vi "Generate AC Measurement Waveform Multi Channel.vi"(6 "hardware commands sync queue":T1, 7 "Voltage(volts)":dbl, 8 "error in":errorcluster, 9 "Frequency":dbl, 10 "DAQmx product name":string, 11 "DSG task in":refnum<k21>) -> (0 "error out":errorcluster, 3 "DSG task out":refnum<k21>)   [LabVIEW 2021, in "audio_adc_acDualChannelMeasurement.lvlib"]
uses:
  audio_adc_acDualChannelMeasurement.lvlib
  shared/controls/Sync Commands Queue Ref.ctl
  shared/controls/Sync Commands.ctl
  <vilib>/addons/_NISVFA/_Generation/Signal Generation/SV Signal/sv_System Timing Model.ctl
  <vilib>/DAQmx/write.llb/DAQmx Write (Analog 1D Wfm NChan NSamp).vi
  <vilib>/addons/_NISVFA/_Generation/Signal Generation/SV Sinusoid/SV Sinusoid.lvclass
  C:/Program Files/National Instruments/LabVIEW 2021/vi.lib/addons/_NISVFA/_Generation/Signal Generation/SV Signal/SV Signal.lvclass
  <vilib>/addons/_NISVFA/_Generation/Signal Generation/SV Sinusoid/Configure Sine.vi
  <vilib>/addons/_NISVFA/_Generation/Signal Generation/SV Signal/Write Sample Rate.vi
  <vilib>/addons/_NISVFA/_Generation/Signal Generation/SV Signal/Write System Timing Model.vi
  <vilib>/addons/_NISVFA/_Generation/Signal Generation/SV Signal/Write Ramp Parameters.vi
  <vilib>/DAQmx/miscellaneous.llb/DAQmx Fill In Error Info.vi
  <resource>/objmgr/daqmx.rc
  <vilib>/addons/_NISVFA/_Generation/Signal Generation/SV Signal/SV Signal.lvclass
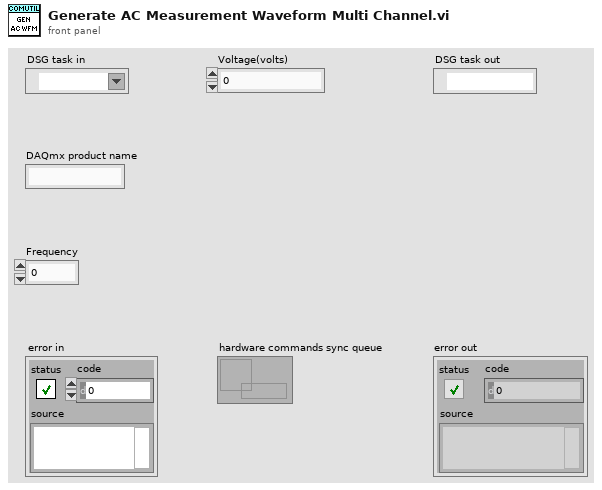
[diagram p1: front panel]
types:
  T1 = typedef "Sync Commands Queue Ref.ctl" = refnum<queue>
  T2 = typedef "Sync Commands.ctl" = enum16{"NoAction", "GenerationStarted", "AcquisitionCompleted", "GenerationErrored"}
  T3 = cluster{"profile":enum16{"Linear", "Half cosine"}, "durations [s]":cluster{"ramp-up":dbl, "transition":dbl, "ramp-down":dbl}}
  T4 = typedef "SV Signal.lvclass/sv_System Timing Model.ctl" = i64
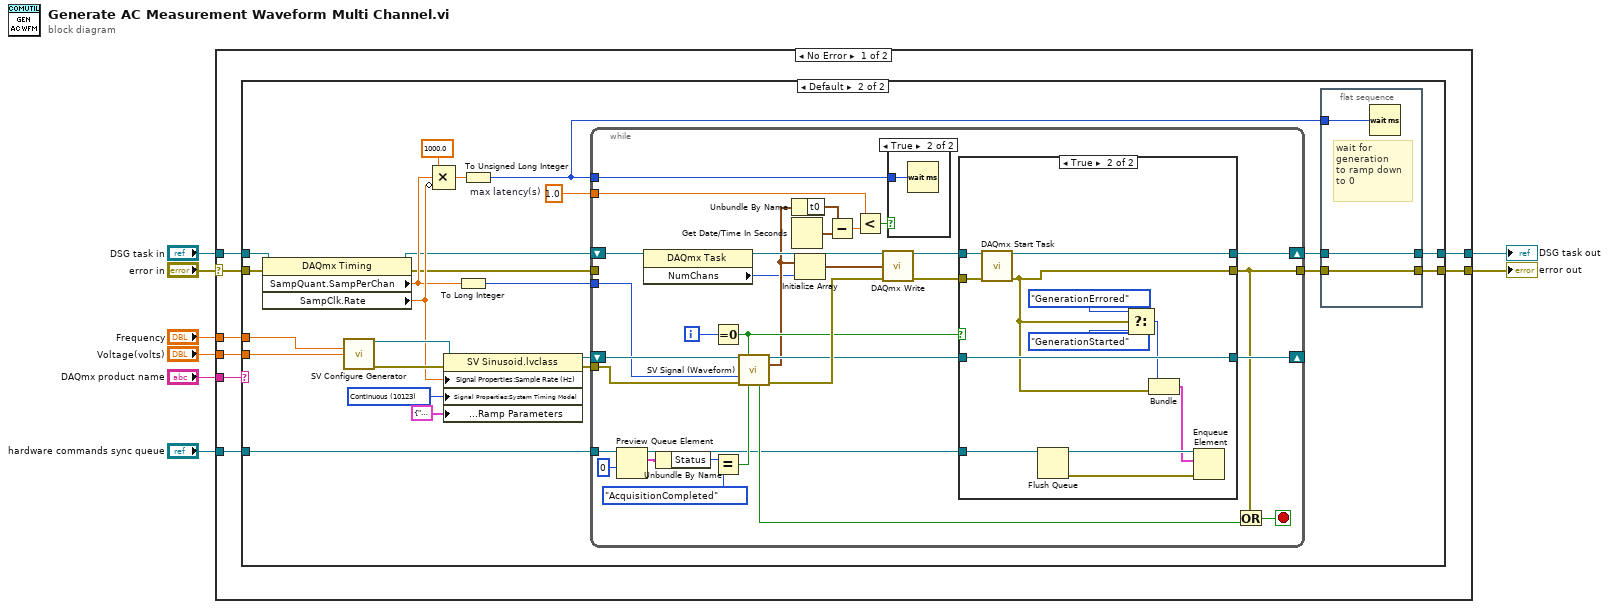
[diagram p0: block diagram]
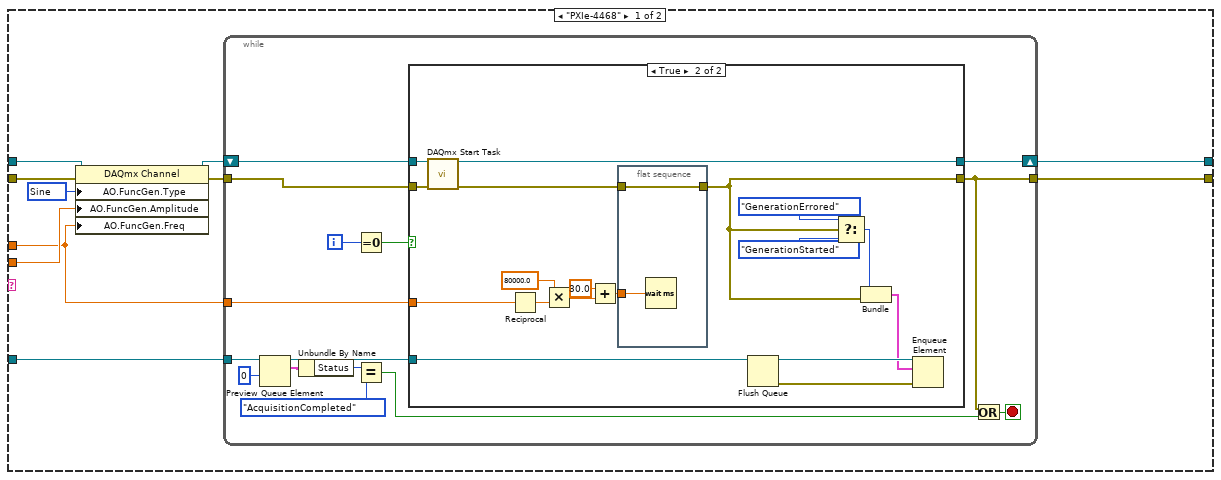
[diagram p2: hidden frame]
diagram:
  n1 = case shown="No Error" "error in" {
    selector: "error in" -> [w16 w140]
    tunnel: [w15 w139] -> w7
    tunnel: [w14 w140] -> w6
    tunnel: "DSG task in" -> [w11 w139]
    tunnel: "hardware commands sync queue" -> [w13 _]
    tunnel: "DAQmx product name" -> [w10 _]
    tunnel: "Frequency" -> [w9 _]
    tunnel: "Voltage(volts)" -> [w12 _]
    frame No Error {
      n2 = case shown="Default" w10 {
        tunnel: w16 -> [w20 w87]
        tunnel: w11 -> [w22 w83]
        tunnel: [w25 w71] -> w15
        tunnel: [w24 w70] -> w14
        tunnel: w13 -> [w26 w68]
        tunnel: w9 -> [w17 w66]
        tunnel: w12 -> [w18 w65]
        frame "PXIe-4468" {
          w19 = 14751 items=["Sine"=14751, "Triangle"=14752, "Square"=14753, "Sawtooth"=14754] ("AO.FuncGen.Type")
          n3 = property class="DAQmx Channel"(reference=w22, error in=w20, "AO.FuncGen.Type"=w19, "AO.FuncGen.Amplitude"=w18, "AO.FuncGen.Freq"=w17) -> (reference out=w23:refnum<k21>, error out=w21:errorcluster)
          n4 = while {
            tunnel: w21 -> [w40]
            shift-right: [w34] -> w25
            shift-left: w23 -> [w39]
            tunnel: [w27] -> w24
            tunnel: w26 -> [w31]
            tunnel: w17 -> [w28]
            i -> [w41]
            stop <- w38 stop-if-true
            n5 = Preview Queue Element(queue=w31, timeout in ms (-1)=0) -> (queue out=w35:T1, element=w33:cluster{"Status":T2, "Error":errorcluster})  [unwired: 1 in, 2 out]
            n6 = Unbundle By Name(w33) -> ("Status"=w32:T2)
            n7 = Equal To 0?(x=w41) -> (x = 0?=w30:bool)
            n8 = Equal?(x=w32, y=Sync_Commands."AcquisitionCompleted") -> (x = y?=w29:bool)
            n9 = case shown="True" w30 {
              tunnel: w35 -> [_ w61]
              tunnel: w39 -> [w43 w59]
              tunnel: [w43 w45] -> w34
              tunnel: w40 -> [w42 w58]
              tunnel: [w42 w47] -> w27
              tunnel: w28 -> [_ w44]
              frame False {
              }
              frame True {
                n10 = call <vilib>:"DAQmx Start Task.vi"("task/channels in"=w59, "error in"=w58) -> ("task out"=w45:refnum<k21>, "error out"=w48:errorcluster)  [unwired: 12 in]
                n11 = Reciprocal(x=w44) -> (1/x=w49:dbl)
                n12 = Multiply(x=80000.0, y=w49) -> (x*y=w51:dbl)
                n13 = Add(x=30.0, y=w51) -> (x+y=w46:dbl)
                n14 = flat-sequence {
                  tunnel: w48 -> [w63]
                  tunnel: [w63] -> w47
                  tunnel: w46 -> [w62]
                  frame #0 {
                    n15 = Wait (ms)(milliseconds to wait=w62) -> ()  [unwired: 1 out]
                  }
                }
                n16 = Flush Queue(queue=w61) -> (queue out=w60:T1, error out=w57:errorcluster)  [unwired: 1 in, 1 out]
                n17 = Select(t=Sync_Commands."GenerationErrored" ("element"), s=w47, f=Sync_Commands."GenerationStarted" ("element")) -> (s? t:f=w54:T2)
                n18 = Bundle("element"=w54, "error out"=w47) -> (w53:cluster{"element":T2, "error out":errorcluster})  [unwired: 1 in]
                n19 = Enqueue Element(queue=w60, element=w53, error in (no error)=w57) -> ()  [unwired: 1 in, 3 out]
              }
            }
            n20 = Or(x=w27, y=w29) -> (x .or. y?=w38:bool)
          }
        }
        frame Default {
          w76 = 1.0  # max latency(s)
          w84 = T4 10123 items=["Finite"=10178, "-"=-1, "Continuous"=10123, "-"=-2, "Settled"=110123, "Averaged"=210123, "Discrete Sweep"=310123, "Continuous Sweep"=410123] ("System Timing Model")
          n21 = property class="DAQmx Timing"(reference=w83, error in=w87) -> (reference out=w77:refnum<k21>, error out=w64:errorcluster, "SampQuant.SampPerChan"=w79:dbl, "SampClk.Rate"=w82:dbl)
          n22 = call-poly <vilib>:"SV Configure Generator.vi"("frequency (Hz)"=w66, "amplitude"=w65) -> ("signal configuration"=w85:refnum<class "SV Sinusoid.lvclass">, "error out"=w86:errorcluster)  [unwired: 12 in]
          n23 = Compound Arithmetic op=MULTIPLY(1000.0 ("value"), w79, invert w82) -> (w75:dbl)
          n24 = property class="SV Sinusoid.lvclass"(reference=w85, error in=w86, "Signal Properties:Sample Rate (Hz)"=w82, "Signal Properties:System Timing Model"=w84, "Signal Properties:Ramps:Ramp Parameters"=T3 {"profile"=enum."Linear", "durations [s]"={"ramp-up"=0.0, "transition"=0.0, "ramp-down"=0.01}} ("Ramp Parameters:All Elements")) -> (reference out=w81:refnum<class "SV Sinusoid.lvclass">, error out=w80:errorcluster)
          n25 = To Long Integer(number=w79) -> (32bit integer=w78:i32)
          n26 = To Unsigned Long Integer(number=w75) -> (unsigned 32bit integer=w69:u32)
          n27 = while {
            shift-right: [w98] -> _
            shift-left: w81 -> [w122]
            tunnel: w80 -> [w119]
            tunnel: w78 -> [w120]
            shift-right: [w101] -> w72
            shift-left: w77 -> [w118]
            tunnel: [w95] -> w73
            tunnel: w76 -> [w111]
            tunnel: w69 -> [w109]
            tunnel: w68 -> [w108]
            tunnel: w64 -> [_]
            i -> [w121]
            stop <- w115 stop-if-true
            n28 = Preview Queue Element(queue=w108, timeout in ms (-1)=0) -> (queue out=w104:T1, element=w97:cluster{"Status":T2, "Error":errorcluster})  [unwired: 1 in, 2 out]
            n29 = property class="DAQmx Task"(reference=w118) -> (reference out=w94:refnum<k21>, "NumChans"=w92:u32)  [unwired: 1 in, 1 out]
            n30 = Unbundle By Name(w97) -> ("Status"=w96:T2)
            n31 = Equal To 0?(x=w121) -> (x = 0?=w103:bool)
            n32 = Equal?(x=w96, y=Sync_Commands."AcquisitionCompleted") -> (x = y?=w105:bool)
            n33 = call-dynamic "SV Signal (Waveform).vi"("signal configuration"=w122, "reset"=w103, "samples"=w120, "error in (no error)"=w119, "stop"=w105) -> ("signal configuration"=w99:refnum<class "SV Sinusoid.lvclass">, "output waveform"=w93:waveform(dbl), "done"=w116:bool, "error out"=w117:errorcluster)  [unwired: 5 in, 2 out]
            n34 = Unbundle By Name(w93) -> ("t0"=w114:timestamp)
            n35 = Get Date/Time In Seconds() -> (seconds since 1Jan1904=w113:timestamp)
            n36 = Initialize Array(w93, w92) -> (w91:waveform(dbl)[])
            n37 = Subtract(x=w114, y=w113) -> (x-y=w112:dbl)
            n38 = Less?(x=w111, y=w112) -> (x < y?=w110:bool)
            n39 = call-poly <vilib>:"DAQmx Write.vi"("task/channels in"=w94, "data"=w91, "error in"=w117) -> ("task out"=w102:refnum<k21>, "error out"=w100:errorcluster)  [unwired: 10 in, 1 out]
            n40 = case shown="True" w110 {
              tunnel: w109 -> [_ w138]
              frame False {
              }
              frame True {
                n41 = Wait (ms)(milliseconds to wait=w138) -> ()  [unwired: 1 out]
              }
            }
            n42 = case shown="True" w103 {
              tunnel: w104 -> [_ w137]
              tunnel: w102 -> [w125 w135]
              tunnel: [w125 w134] -> w101
              tunnel: w100 -> [w124 w133]
              tunnel: [w124 w127] -> w95
              tunnel: w99 -> [w123 w129]
              tunnel: [w123 w129] -> w98
              frame False {
              }
              frame True {
                n43 = call <vilib>:"DAQmx Start Task.vi"("task/channels in"=w135, "error in"=w133) -> ("task out"=w134:refnum<k21>, "error out"=w127:errorcluster)  [unwired: 12 in]
                n44 = Flush Queue(queue=w137) -> (queue out=w136:T1, error out=w132:errorcluster)  [unwired: 1 in, 1 out]
                n45 = Select(t=Sync_Commands."GenerationErrored" ("element"), s=w127, f=Sync_Commands."GenerationStarted" ("element")) -> (s? t:f=w128:T2)
                n46 = Bundle("element"=w128, "error out"=w127) -> (w126:cluster{"element":T2, "error out":errorcluster})  [unwired: 1 in]
                n47 = Enqueue Element(queue=w136, element=w126, error in (no error)=w132) -> ()  [unwired: 1 in, 3 out]
              }
            }
            n48 = Or(x=w95, y=w116) -> (x .or. y?=w115:bool)
          }
          n49 = flat-sequence {
            tunnel: w73 -> [w89]
            tunnel: w72 -> [w90]
            tunnel: [w90] -> w71
            tunnel: [w89] -> w70
            tunnel: w69 -> [w88]
            frame #0 {
              # "wait for\ngeneration\nto ramp down\nto 0"
              n50 = Wait (ms)(milliseconds to wait=w88) -> ()  [unwired: 1 out]
            }
          }
        }
      }
    }
    frame Error {
    }
  }
  "DSG task out" <- w7
  "error out" <- w6
